vi "IIR Filter.vi"(0 "Neural, z":dbl[](array[numeric]) format="%.3f", 1 "Outputs, P":i32=1 min=1 max=10 step=1, 2 "Total control, U":dbl=1.0 min=1.0 max=10.0 step=1.0 format="%.3f", 3 "Persistant signal, ps":dbl format="%.2e", 4 "Wavenet-IIR Values":T1 {"Function, dy" format="%.3f"; "Function, y" format="%.3f"; "Tau, t" format="%.3f"; "Forwards, D" format="%.3f"; "Feedbacks, C" format="%.3f"; "Weights, W" format="%.3f"; "Shifts, B" format="%.3f"; "Scales, A" format="%.3f"}, 5 "Wavenet-IIR Memories":T3 {"Activation functions, dF" format="%.3f"; "Wavenet, Z" format="%.3f"; "Tracking errors, e" format="%.3f"; "Activation functions, F" format="%.3f"; "Wavenet-IIR, Y" format="%.3f"}) -> (6 "Wavenet-IIR Outputs":T2 {"Rho, R" format="%.3f"; "Gamma, G" format="%.3f"; "Estimated, y" format="%.3f"; "Neural, z" format="%.3f"})   [LabVIEW 2022 SP3]
uses:
  <vilib>/Analysis/baseanly.llb/Real A x B.vi
  <vilib>/Analysis/Matrix/Numeric/Multiply/Multiply - R,RM.vi
  <vilib>/Analysis/NI_AALBase.lvlib
  <vilib>/Analysis/Matrix/NI_Matrix.lvlib
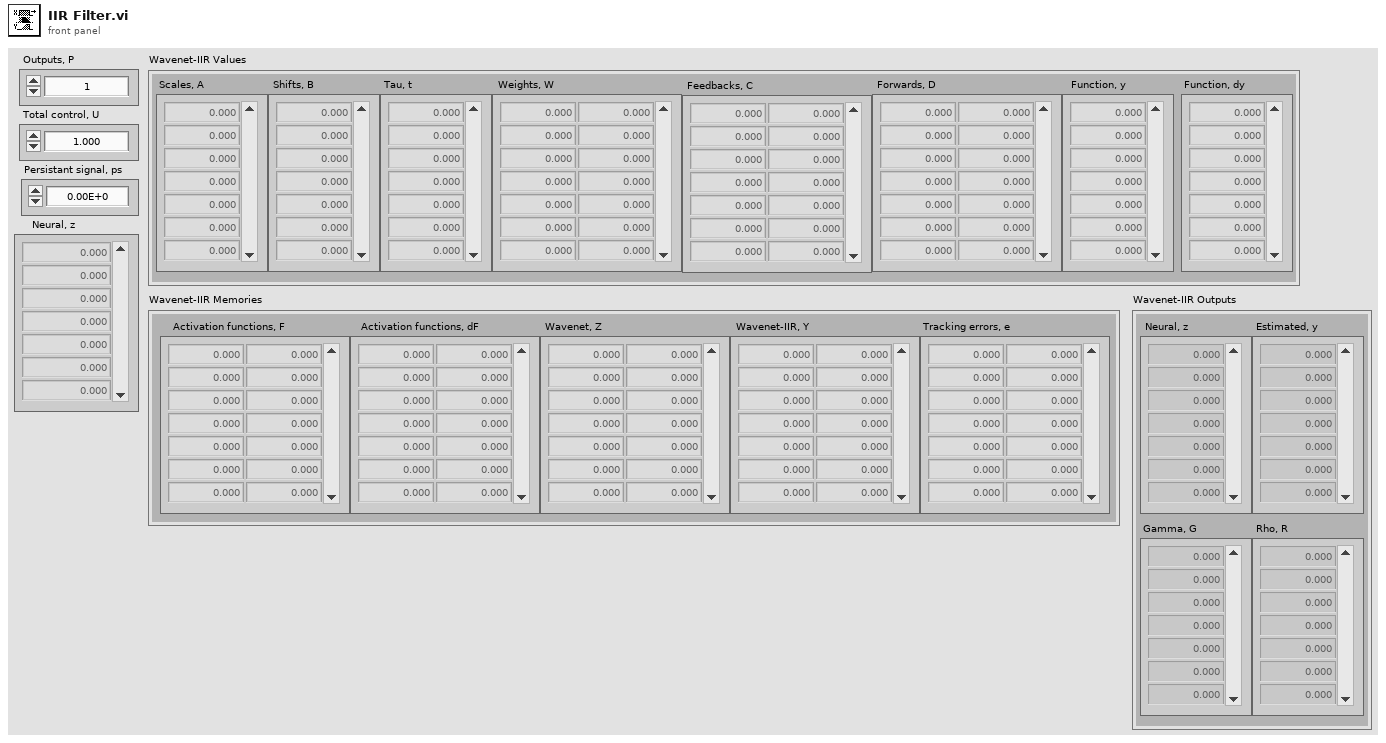
[diagram p1: front panel]
types:
  T1 = cluster{"Scales, A":dbl[], "Shifts, B":dbl[], "Weights, W":dbl[][], "Feedbacks, C":dbl[][], "Forwards, D":dbl[][], "Tau, t":dbl[], "Function, y":dbl[], "Function, dy":dbl[]}
  T2 = cluster{"Neural, z":dbl[], "Estimated, y":dbl[], "Gamma, G":dbl[], "Rho, R":dbl[]}
  T3 = cluster{"Wavenet-IIR, Y":dbl[][], "Activation functions, F":dbl[][], "Tracking errors, e":dbl[][], "Wavenet, Z":dbl[][], "Activation functions, dF":dbl[][]}
  T4 = typedef "NI_Matrix.lvlib/RealMatrix.ctl" = dbl[][]
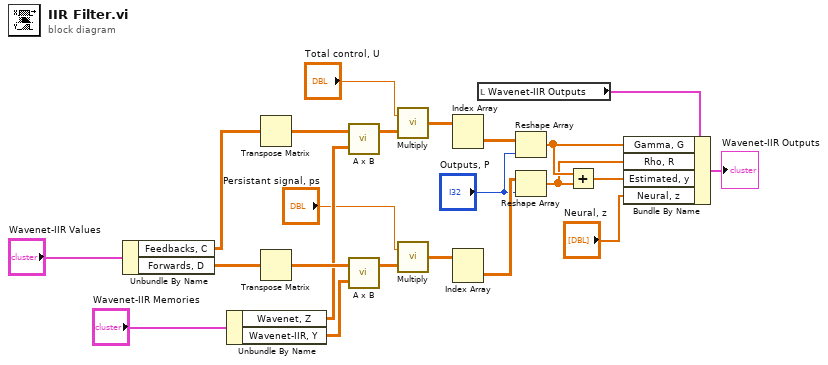
[diagram p0: block diagram]
diagram:
  n1 = Unbundle By Name("Wavenet-IIR Values") -> ("Feedbacks, C"=w18:dbl[][], "Forwards, D"=w22:dbl[][])
  n2 = Unbundle By Name("Wavenet-IIR Memories") -> ("Wavenet, Z"=w20:dbl[][], "Wavenet-IIR, Y"=w23:dbl[][])
  n3 = Transpose Matrix(1:w18) -> (0:w19:dbl[][])
  n4 = Transpose Matrix(1:w22) -> (0:w21:dbl[][])
  n5 = call-poly <vilib>:"A x B.vi"("B"=w20, "A"=w19) -> ("A x B"=w14:T4)  [unwired: 1 out]
  n6 = call-poly <vilib>:"A x B.vi"("B"=w23, "A"=w21) -> ("A x B"=w12:T4)  [unwired: 1 out]
  n7 = call-poly <vilib>:"Multiply.vi"("Real Matrix A"=w14, "Real Scalar c"="Total control, U") -> ("c * A"=w11:T4)
  n8 = call-poly <vilib>:"Multiply.vi"("Real Matrix A"=w12, "Real Scalar c"="Persistant signal, ps") -> ("c * A"=w9:T4)
  n9 = Index Array(array=w11) -> (element=w5:T4)  [unwired: 2 in]
  n10 = Index Array(array=w9) -> (element=w8:T4)  [unwired: 2 in]
  n11 = local read "Wavenet-IIR Outputs"() -> (w10:T2)
  n12 = Reshape Array(w5, "Outputs, P") -> (w3:dbl[])
  n13 = Reshape Array(w8, "Outputs, P") -> (w2:dbl[])
  n14 = Add(x=w3, y=w2) -> (x+y=w1:dbl[])
  n15 = Bundle By Name(cluster=w10, "Gamma, G"=w3, "Rho, R"=w2, "Estimated, y"=w1, "Neural, z"="Neural, z") -> (→"Wavenet-IIR Outputs":T2)
